vi "SourceSet.vi"(3 "Source":string="PI1-MAGLITE", 4 "Intensity":i32, 9 "error in (no error)":errorcluster) -> (0 "Source out":string="PI1-MAGLITE", 1 "Ok?":refnum<k4>, 6 "error out":errorcluster)   [LabVIEW 2009]
uses:
  Controls/SourceCommand.ctl
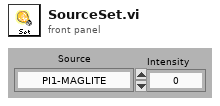
[diagram p1: front panel]
types:
  T1 = typedef "SourceCommand.ctl" = cluster{"Source":string, "Command":enum16{"INTENSITY", "ALL OFF", "QUIT"}, "Intensity":i32, "Ok?":refnum<k4>}
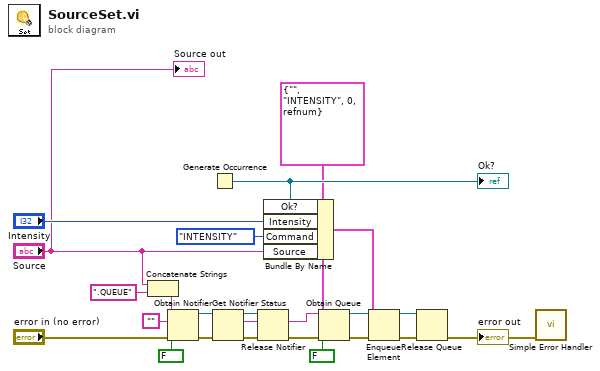
[diagram p0: block diagram]
diagram:
  w15 = T1 {"Source"="", "Command"=enum."INTENSITY", "Intensity"=0, "Ok?"=refnum} ("SourceCommand")
  n1 = Concatenate Strings("Source", ".QUEUE") -> (w9:string)
  n2 = Obtain Notifier(name (unnamed)=w9, notification data type="", create if not found? (T)=FALSE ("créer si introuvable ? (T)"), error in (no error)="error in (no error)") -> (notifier out=w10:refnum<notifier>, error out=w11:errorcluster)  [unwired: 1 out]
  n3 = Generate Occurrence() -> (w17:refnum<k4>)
  "Ok?" <- w17
  n4 = Get Notifier Status(notifier=w10, error in (no error)=w11) -> (notifier out=w13:refnum<notifier>, current notification=w2:string, error out=w14:errorcluster)  [unwired: 2 out]
  n5 = Release Notifier(notifier=w13, error in (no error)=w14) -> (error out=w5:errorcluster)  [unwired: 3 out]
  n6 = Bundle By Name(cluster=w15, "Ok?"=w17, "Intensity"="Intensity", "Command"=enum16{"INTENSITY", "ALL OFF", "QUIT"}."INTENSITY", "Source"="Source") -> (w21:T1)
  n7 = Obtain Queue(name (unnamed)=w2, element data type=w15, create if not found? (T)=FALSE ("créer si introuvable ? (T)"), error in (no error)=w5) -> (queue out=w23:refnum<queue>, error out=w22:errorcluster)  [unwired: 1 in, 1 out]
  n8 = Enqueue Element(queue=w23, element=w21, error in (no error)=w22) -> (queue out=w19:refnum<queue>, error out=w20:errorcluster)  [unwired: 2 out]
  n9 = Release Queue(queue=w19, error in (no error)=w20) -> (error out=w1:errorcluster)  [unwired: 3 out]
  "error out" <- w1
  n10 = call <vilib>:"Simple Error Handler.vi"("error in (no error)"=w1) -> ()  [unwired: 1 in, 8 out]
  "Source out" <- "Source"
